vi "FGA Find Waypoint With Id.vi"(0 "Element UID":u16) -> (1 "Record Exists?":bool, 2 "Component Index":i32, 3 "ElementRec":T1)   [LabVIEW 2009]
uses:
  LocalWaypointRec.ctl
  ElementRec.ctl
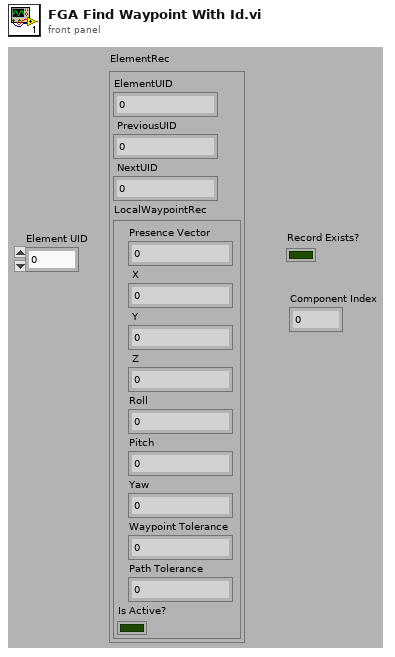
[diagram p1: front panel]
types:
  T1 = typedef "ElementRec.ctl" = cluster{"ElementUID":u16, " PreviousUID":u16, " NextUID":u16, "LocalWaypointRec":T2}
  T2 = typedef "LocalWaypointRec.ctl" = cluster{"Presence Vector":u8, " X":dbl, " Y":dbl, " Z":dbl, "Roll":dbl, "Pitch":dbl, "Yaw":dbl, "Waypoint Tolerance":dbl, "Path Tolerance":dbl, "Is Active?":bool}
  T3 = typedef "ElementRec.ctl" = cluster{"ElementUID":u16, " PreviousUID":u16, " NextUID":u16, "Presence Vector":u8, "LocalWaypointRec":T4}
  T4 = typedef "LocalWaypointRec.ctl" = cluster{" X":dbl, " Y":dbl, " Z":dbl, "Roll":dbl, "Pitch":dbl, "Yaw":dbl, "Waypoint Tolerance":dbl, "Path Tolerance":dbl, "Is Active":bool}
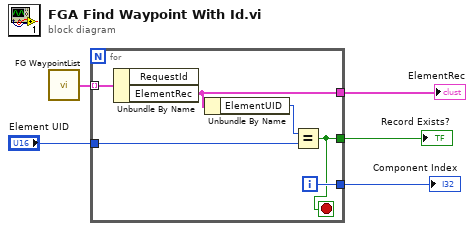
[diagram p0: block diagram]
diagram:
  n1 = call "FG WaypointList.vi"() -> ("Local Waypoint List out"=w5:T1[])  [unwired: 2 in]
  n2 = for {
    tunnel: w5 -> [w11] mode=indexing
    tunnel: "Element UID" -> [w10]
    tunnel: [w6] -> w3
    tunnel: [w8] -> w2
    tunnel: [w7] -> w1
    i -> [w7]
    stop <- w6 stop-if-true
    n3 = Unbundle By Name(w11) -> ("ElementRec"=w8:T3)  [unwired: 1 out]
    n4 = Unbundle By Name(w8) -> ("ElementUID"=w9:u16)
    n5 = Equal?(x=w9, y=w10) -> (x = y?=w6:bool)
  }
  "Record Exists?" <- w3
  "ElementRec" <- w2
  "Component Index" <- w1
